vi "Move Splitters.vi"(4 "Old Width":i16, 6 "New Width":i16, 8 "error in":errorcluster, 11 "Left Splitter":refnum<vi>) -> (0 "error out":errorcluster)   [LabVIEW 2020]
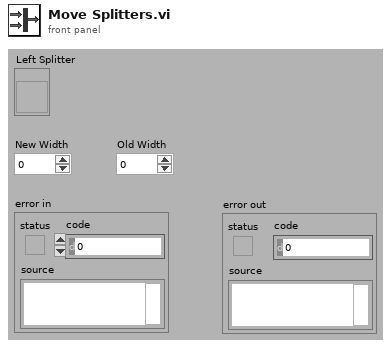
[diagram p1: front panel]
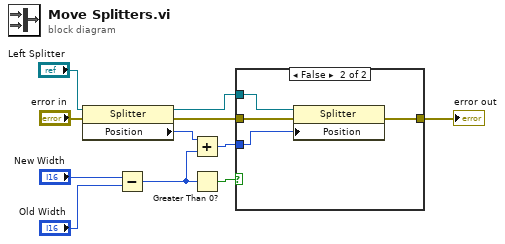
[diagram p0: block diagram]
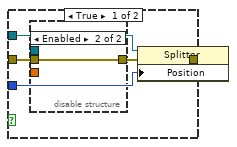
[diagram p2: hidden frame]
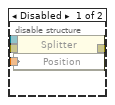
[diagram p3: hidden frame]
diagram:
  n1 = property class="Splitter"(reference="Left Splitter", error in="error in") -> (reference out=w4:refnum<vi>, error out=w2:errorcluster, "Position"=w6:i32)
  n2 = Subtract(x="New Width", y="Old Width") -> (x-y=w1:i16)
  n3 = Add(x=w6, y=w1) -> (x+y=w7:i32)
  n4 = Greater Than 0?(x=w1) -> (x > 0?=w8:bool)
  n5 = case shown="False" w8 {
    tunnel: w2 -> [w16 w23]
    tunnel: w4 -> [w15 w25]
    tunnel: w7 -> [w14 w24]
    tunnel: [w12 w22] -> w9
    frame True {
      n6 = disable-structure shown="Enabled" {
        disable-tunnel: w16 -> [w20 w21]
        disable-tunnel: _ -> [w19 _]
        disable-tunnel: _ -> [w18 _]
        disable-tunnel: [w17 w21] -> w13
        frame Disabled {
          n7 = property class="Splitter"(reference=w19, error in=w20, "Position"=w18) -> (error out=w17:errorcluster)  [unwired: 1 out]
        }
        frame Enabled {
        }
      }
      n8 = property class="Splitter"(reference=w15, error in=w13, "Position"=w14) -> (error out=w12:errorcluster)  [unwired: 1 out]
    }
    frame False {
      n9 = property class="Splitter"(reference=w25, error in=w23, "Position"=w24) -> (error out=w22:errorcluster)  [unwired: 1 out]
    }
  }
  "error out" <- w9
